vi "GetPath_Dialog.vi"() -> (1 "Cancelled?":bool, 3 "File Paths Out":T1)   [LabVIEW 2009]
uses:
  typedefs/PathCluster.ctl
panel:
  in  "Cancel":bool
  in  "OK":bool
  in  "File Paths":T1
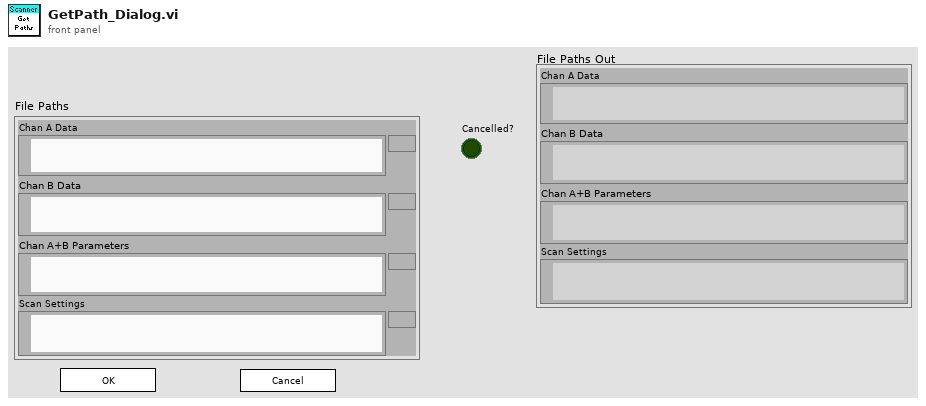
[diagram p1: front panel]
types:
  T1 = typedef "PathCluster.ctl" = cluster{"Chan A Data":path, "Chan B Data":path, "Chan A+B Parameters":path, "Scan Settings":path}
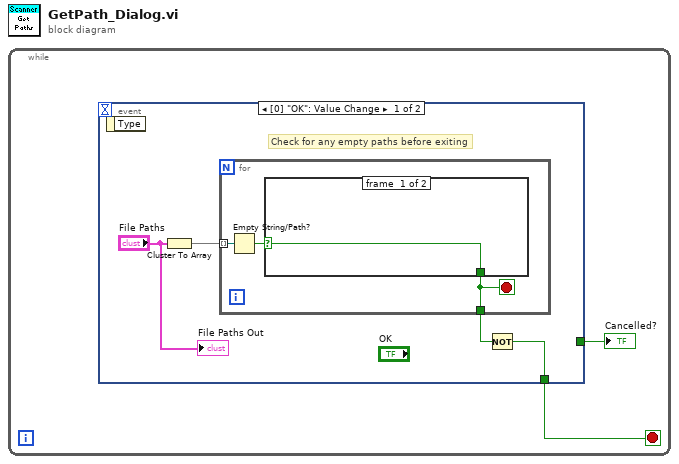
[diagram p0: block diagram]
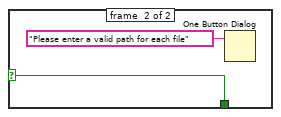
[diagram p2: hidden frame]
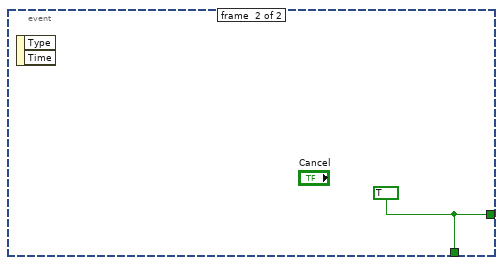
[diagram p3: hidden frame]
diagram:
  n1 = while {
    stop <- w2 stop-if-true
    n2 = event shown="[0] \"OK\": Value Change" {
      selector: _ -> [_ _]
      dyn-events: _ -> [_ _]
      timeout: _ -> [_ _]
      tunnel: [w4 w13] -> w2
      tunnel: [_ w13] -> w1
      event #0 {
        # "Check for any empty paths before exiting"
        n3 = event-data() -> ()  [unwired: 1 in, 1 out]
        n4 = Cluster To Array(cluster="File Paths") -> (array=w6:path[])
        n5 = for {
          tunnel: w6 -> [w9] mode=indexing
          tunnel: [w7] -> w5
          stop <- w7 stop-if-true
          n6 = Empty String/Path?(string/path=w9) -> (empty?=w8:bool)
          n7 = case shown="False" w8 {
            selector: w8 -> [w10 w11]
            tunnel: [w10 w11] -> w7
            frame #0 {
            }
            frame #1 {
              n8 = One Button Dialog(message="Please enter a valid path for each file") -> ()  [unwired: 1 in, 1 out]
            }
          }
        }
        n9 = Not(x=w5) -> (.not. x?=w4:bool)
        "File Paths Out" <- "File Paths"
      }
      event #1 {
        w13 = TRUE ("OK")
        n10 = event-data() -> ()  [unwired: 1 in, 2 out]
      }
    }
    "Cancelled?" <- w1
  }
